vi "Create or Write Workbook.vi"(8 "error in (no error)":errorcluster, 10 "File Name":path, 11 "IWorkbook Reference":refnum<k24>) -> (0 "error out":errorcluster, 3 "IWorkbook Reference Out":refnum<k24>)   [LabVIEW 2014]
uses:
  C:/Users/LENOVO/Desktop/CodeSpace GUI/LVExcel/Resources/net40/NPOI.dll
  Resources/net40/NPOI.dll
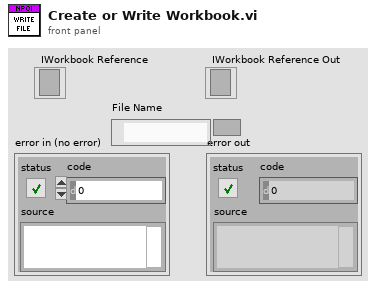
[diagram p1: front panel]
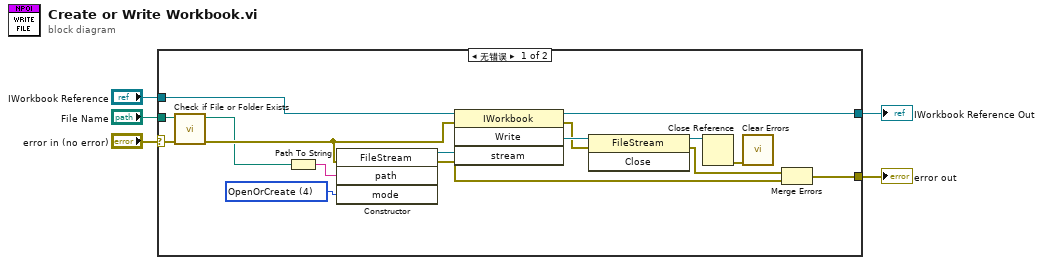
[diagram p0: block diagram]
diagram:
  n1 = case shown="无错误" "error in (no error)" {
    selector: "error in (no error)" -> [w14 w22]
    tunnel: "IWorkbook Reference" -> [w20 w21]
    tunnel: [w19 w21] -> w4
    tunnel: [w18 w22] -> w3
    tunnel: "File Name" -> [w16 _]
    frame No Error {
      w12 = 4 items=["CreateNew"=1, "Create"=2, "Open"=3, "OpenOrCreate"=4, "Truncate"=5, "Append"=6] ("mode")
      n2 = call <vilib>:"Check if File or Folder Exists.vi"("error in (no error)"=w14, "path"=w16) -> ("error out"=w17:errorcluster, "dup path"=w15:path)  [unwired: 7 in, 1 out]
      n3 = Path To String(path=w15) -> (string=w13:string)
      n4 = constructor class="FileStream"(error in=w17, "path"=w13, "mode"=w12) -> (reference out=w9:refnum<k24>, error out=w11:errorcluster)  [unwired: 2 in, 3 out]
      n5 = invoke class="IWorkbook" method="Write"(reference=w20, error in=w17, "stream"=w9) -> (reference out=w19:refnum<k24>, error out=w7:errorcluster)  [unwired: 1 in, 2 out]
      n6 = invoke class="FileStream" method="Close"(reference=w9, error in=w7) -> (reference out=w8:refnum<k24>, error out=w6:errorcluster)  [unwired: 1 in, 1 out]
      n7 = Close Reference(reference=w8) -> (error out=w10:errorcluster)  [unwired: 1 in]
      n8 = call <vilib>:"Clear Errors.vi"("error in (no error)"=w10) -> ()  [unwired: 5 in, 2 out]
      n9 = Merge Errors(w6, w11) -> (w18:errorcluster)
    }
    frame Error {
    }
  }
  "IWorkbook Reference Out" <- w4
  "error out" <- w3
